vi "Process_Replace.vi"(4 "Index":i32, 6 "Replace array":string[](array[string]), 7 "Array In":string[][](array[string])) -> (3 "Array Out":string[][](array[string]))   [LabVIEW 2020]
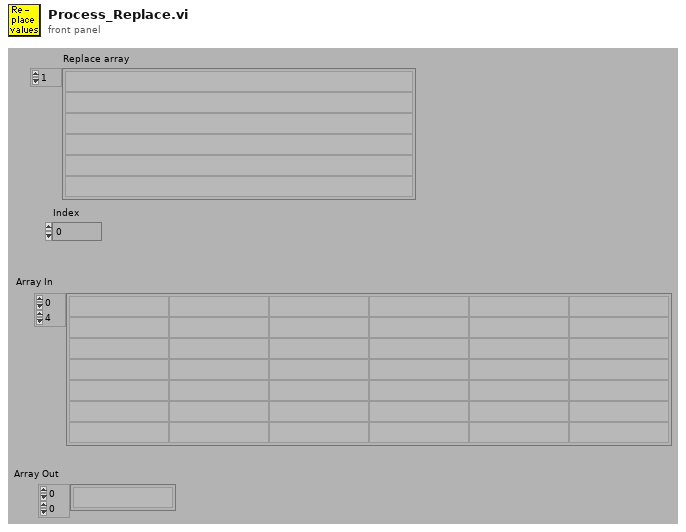
[diagram p1: front panel]
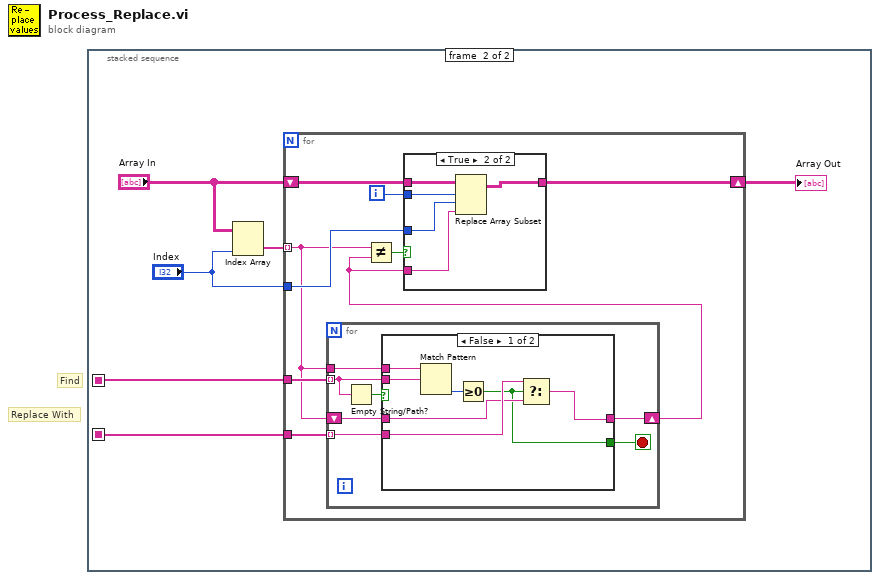
[diagram p0: block diagram]
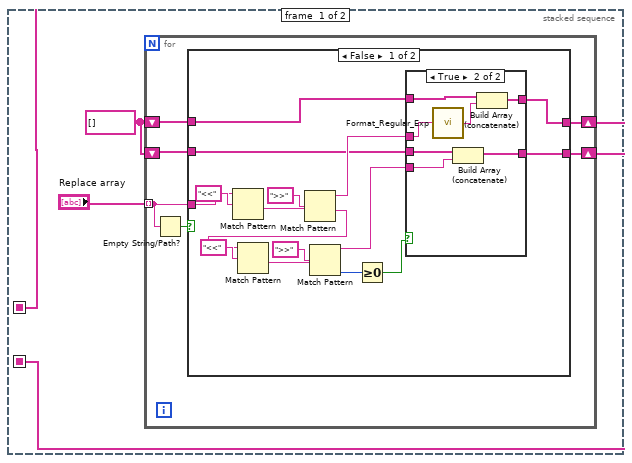
[diagram p2: hidden frame]
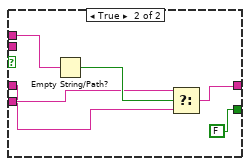
[diagram p5: hidden frame]
diagram:
  # "Replace With"
  # "Find"
  n1 = stacked-sequence {
    seq-local: [w2 _] -> [_ w42]
    seq-local: [w1 _] -> [_ w41]
    frame #0 {
      w3 = string[] []
      n2 = for {
        tunnel: "Replace array" -> [w10] mode=indexing
        shift-right: [w7] -> w2
        shift-left: w3 -> [w8]
        shift-right: [w5] -> w1
        shift-left: w3 -> [w6]
        n3 = Empty String/Path?(string/path=w10) -> (empty?=w9:bool)
        n4 = case shown="False" w9 {
          tunnel: w10 -> [w25 _]
          tunnel: w8 -> [w18 w36]
          tunnel: [w17 w36] -> w7
          tunnel: w6 -> [w15 w37]
          tunnel: [w13 w37] -> w5
          frame False {
            n5 = Match Pattern(string=w25, regular expression="<<") -> (after substring=w24:string)  [unwired: 4 out]
            n6 = Match Pattern(string=w24, regular expression=">>") -> (before substring=w16:string, after substring=w19:string)  [unwired: 3 out]
            n7 = Match Pattern(string=w19, regular expression="<<") -> (after substring=w21:string)  [unwired: 4 out]
            n8 = Match Pattern(string=w21, regular expression=">>") -> (before substring=w14:string, offset past match=w12:i32)  [unwired: 3 out]
            n9 = Greater Or Equal To 0?(x=w12) -> (x >= 0?=w11:bool)
            n10 = case shown="True" w11 {
              tunnel: w18 -> [w28 w35]
              tunnel: [w28 w34] -> w17
              tunnel: w16 -> [_ w30]
              tunnel: w15 -> [w27 w33]
              tunnel: w14 -> [_ w32]
              tunnel: [w27 w31] -> w13
              frame False {
              }
              frame True {
                n11 = call "Format_Regular_Exp.vi"("Regular expression"=w30) -> ("Case Insensitive for html"=w29:string)
                n12 = Build Array (concatenate)(w33, w32) -> (w31:string[])
                n13 = Build Array (concatenate)(w35, w29) -> (w34:string[])
              }
            }
          }
          frame True {
          }
        }
      }
    }
    frame #1 {
      n14 = Index Array(array="Array In", index (col)="Index") -> (element=w40:string[])  [unwired: 1 in]
      n15 = for {
        tunnel: w40 -> [w45] mode=indexing
        tunnel: w42 -> [w52]
        tunnel: w41 -> [w51]
        tunnel: "Index" -> [w50]
        shift-right: [w47] -> w38
        shift-left: "Array In" -> [w48]
        i -> [w49]
        n16 = for {
          tunnel: w51 -> [w58] mode=indexing
          tunnel: w52 -> [w55] mode=indexing
          tunnel: w45 -> [w59]
          shift-right: [w57] -> w46
          shift-left: w45 -> [w56]
          stop <- w53 stop-if-true
          n17 = Empty String/Path?(string/path=w55) -> (empty?=w54:bool)
          n18 = case shown="False" w54 {
            tunnel: w55 -> [w66 _]
            tunnel: w59 -> [w65 w72]
            tunnel: w58 -> [w63 w70]
            tunnel: w56 -> [w62 w69]
            tunnel: [w61 w68] -> w57
            tunnel: [w60 FALSE] -> w53
            frame False {
              n19 = Match Pattern(string=w65, regular expression=w66) -> (offset past match=w64:i32)  [unwired: 4 out]
              n20 = Greater Or Equal To 0?(x=w64) -> (x >= 0?=w60:bool)
              n21 = Select(t=w63, s=w60, f=w62) -> (s? t:f=w61:string)
            }
            frame True {
              n22 = Empty String/Path?(string/path=w72) -> (empty?=w71:bool)
              n23 = Select(t=w70, s=w71, f=w69) -> (s? t:f=w68:string)
            }
          }
        }
        n24 = Not Equal?(x=w45, y=w46) -> (x != y?=w44:bool)
        n25 = case shown="True" w44 {
          tunnel: [w73 w75] -> w47
          tunnel: w49 -> [_ w78]
          tunnel: w50 -> [_ w77]
          tunnel: w48 -> [w73 w76]
          tunnel: w46 -> [_ w74]
          frame False {
          }
          frame True {
            n26 = Replace Array Subset(array=w76, new element=w74, index (row)=w78, index (col)=w77) -> (w75:string[][])
          }
        }
      }
      "Array Out" <- w38
    }
  }
